vi "LineAlignment.vi"() -> ()   [LabVIEW 2018]
uses:
  <vilib>/Platform/TimedLoop/XDataNode/timing_clust.ctl
  <vilib>/Platform/TimedLoop/XDataNode/nitl_modes.ctl
  <vilib>/Platform/TimedLoop/XDataNode/wakeup.ctl
  LineAlignNotifier.ctl
  Drive/driveShifterEnum.ctl
  <userlib>/836-Library/System/TDMS_V2/Support/TDMS_DevRef.ctl
  <userlib>/836-Library/System/TDMS_V2/Support/Logging_Settings.ctl
  <userlib>/836-Library/System/TDMS_V2/Support/Group_FIFO_Config.ctl
  <userlib>/836-Library/System/TDMS_V2/Support/Channel_FIFO_Config.ctl
  <vilib>/addons/control/pid/pid.llb/PID (DBL).vi
  <vilib>/platform/TimedLoop/XDataNode/XDataNode.xnode
  <vilib>/addons/control/pid/NI_PID_pid.lvlib
  <vilib>/Platform/TimedLoop/XDataNode/XDNodeRunTimeDep.lvlib
panel:
  in  "Tab Control":enum32{"Auto Tape Alignment", "Drive PID Tune"}(tab)
  out "Chart":cluster{i16, i16, i16, "count":i32, "f":i32}(graph)={0, 0, 0, "count"=0, "f"=4}
  out "Late?":bool
  out "Arrived":bool=TRUE
  in  "Tol (in)":dbl=1.0
  in  "Tol (sec)":dbl=0.35 format="%#_13g"
  out "Right Front":bool
  out "Left Front":bool
  out "Right Rear":bool
  in  "PID gains":T1={"proportional gain (Kc)"=0.014, "integral time (Ti, min)"=0.02, "derivative time (Td, min)"=0.0001} {"derivative time (Td, min)" format="%.8f"; "integral time (Ti, min)" format="%.4f"; "proportional gain (Kc)" format="%.4f"}
  in  "clamp":cluster{"output high":dbl, "output low":dbl}={"output high"=1.0, "output low"=-1.0} {"output low" format="%.2f"; "output high" format="%.2f"}
  in  "Fwd offset Low":dbl=12.0
  in  "Rvs offset Low":dbl=12.0
  out "Goal":dbl=227.0788079155816
  out "Distance":dbl=227.1760531955295
  out "Tape Width":dbl=-5.971765136718773
  out "State":i32=4
  out "Error":dbl=-0.09724527994791288
  out "Count":i32
  out "Period":i64=10
  out "Left Rear":bool
  out "Fire Left":bool=TRUE
  out "Fire Right":bool
  in  "Push Drive":bool
  in  "Tune PID":bool
  in  "lo speed":dbl=0.4 format="%#_13g"
  in  "hi speed":dbl=0.75 format="%#_13g"
  in  "Avg Enc?":bool=TRUE
  in  "dead":dbl=0.05
  in  "Rvs offset High":dbl=12.0
  in  "Fwd offset High":dbl=12.0
  in  "Reset":bool
  in  "Rev":bool
  out "Align Assist":bool
  in  "Set":dbl(slide)=-0.07974481658691701 scale=-50.0..50.0
  in  "output range":cluster{"output high":dbl, "output low":dbl}={"output high"=0.65, "output low"=-0.65} {"output low" format="%.2f"; "output high" format="%.2f"}
  in  "PID gains 2":T1={"proportional gain (Kc)"=0.01, "integral time (Ti, min)"=0.01, "derivative time (Td, min)"=0.0001} {"derivative time (Td, min)" format="%.8f"; "integral time (Ti, min)" format="%.4f"; "proportional gain (Kc)" format="%.4f"}
  out "PID":cluster{"Set":dbl, "Distance":dbl}(graph)={"Set"=95.92025518341308, "Distance"=89.06027364430147}
  out "Error 2":dbl=6.859981539111601
  out "Motor":dbl=0.7000000000000001 format="%.2f"
  in  "reinit?":bool
  in  "negate":bool
  out "Arrived 2":bool
  in  "Tol (in) 2":dbl=0.75
  in  "Tol (sec) 2":dbl=0.35 format="%#_13g"
  out "Enc (in)":dbl=89.06027364430147
  out "Tuning":bool
  in  "Fwd":bool=TRUE
  out "Add":i32=96
  in  "dead 2":dbl=0.05
  in  "Reset Enc":bool
  # "old values;"
  # "Offset for Hi Gear = 21\"\nOffset for Lo Gear = 37\""
  # "Larger values move goal\nfurther in direction of travel"
  # "Diagnostics Only"
  # "Offset for Hi Gear = 12\"\nOffset for Lo Gear = 12\""
  # "2019 P-Bot Hi Gear values:\nP=0.0140, I=0.020, D=0.008"
  # "2019 P-Bot Lo Gear values:\nP=0.0, I=0.0, D=0.0"
  # "Initial 2019 Gear Set"
  # "2019 P-Bot Hi Gear values:\nP=0.0850, I=0.0090, D=0.000,000,08"
  # "2016 C-Bot Bot values:\nP=0.080, I=0.008, D=0.002"
  # "2019 P-Bot Lo Gear values:\nP=0.0350, I=0.0220, D=0.000,400"
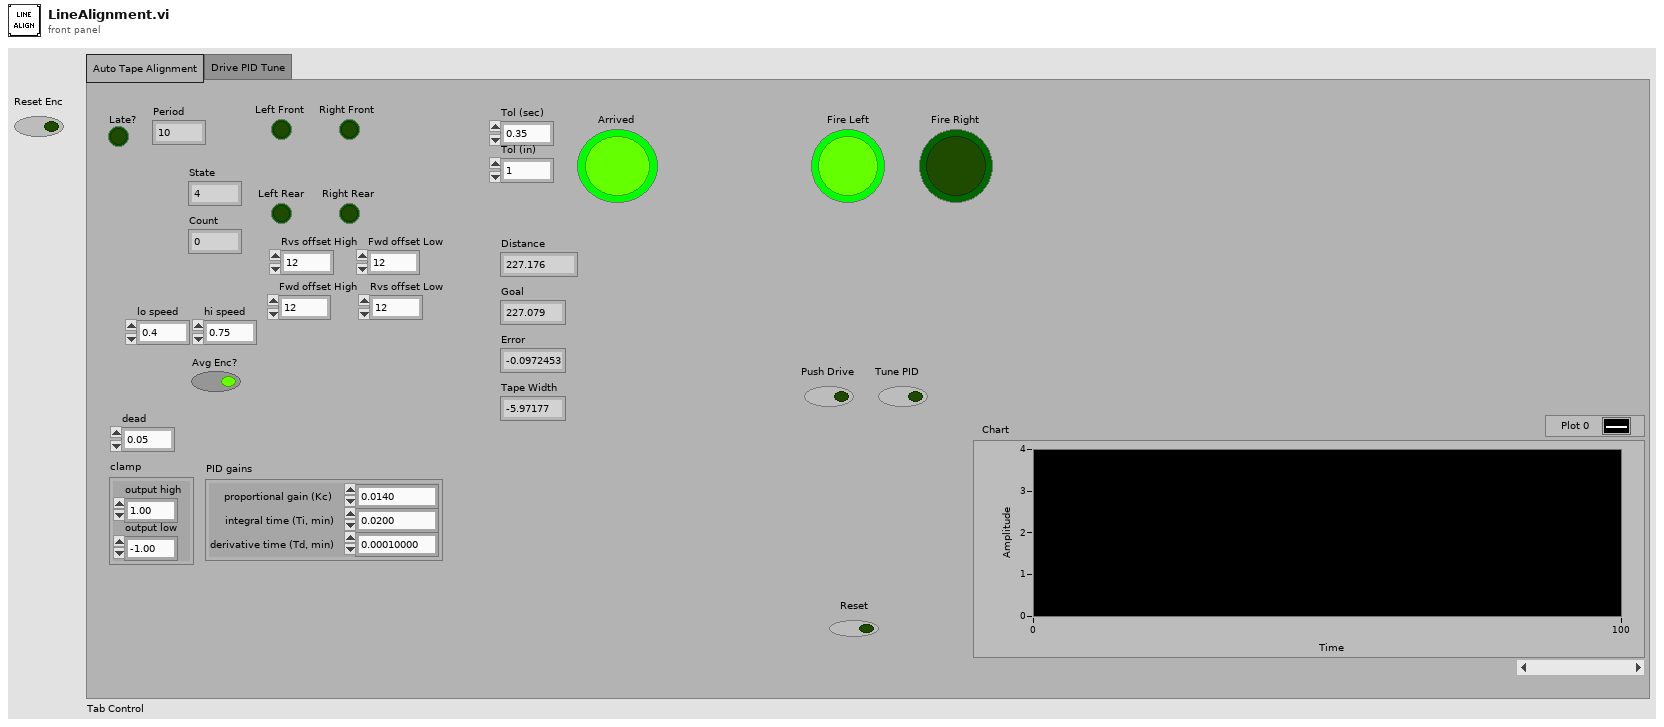
[diagram p1: front panel]
types:
  T1 = cluster{"proportional gain (Kc)":dbl, "integral time (Ti, min)":dbl, "derivative time (Td, min)":dbl}
  T2 = typedef "XDNodeRunTimeDep.lvlib/timing_clust.ctl" = cluster{"Expected End [f-1]":u64, "Actual End [f-1]":u64, "Finished Late? [f-1]":bool, "Expected End [i-1]":u64, "Actual End [i-1]":u64, "Finished Late? [i-1]":bool, "Expected Start [i]":u64, "Actual Start [i]":u64, "Expected Start [f]":u64, "Actual Start [f]":u64, "Source Name":string, "Structure Name":string, "Period":i64, "Deadline":i64, "Offset":i64, "Start":i64, "Priority":i32, "Timeout":i32, "Mode":T3, "Wakeup Reason":T4, "Error":errorcluster, "Source Type":string, "Secondary Source Type":string, "Global End Time":u64, "Global Start Time":u64, "Frame Duration":u64, "Iteration Duration":u64, "Assigned CPU":i32, "I/O Scan Engine Mode":u32}
  T3 = typedef "XDNodeRunTimeDep.lvlib/nitl_modes.ctl" = enum32{"No Change", "Process missed periods, maintain original phase", "Discard missed periods, maintain original phase", "Process missed periods, ignore original phase", "Discard missed periods, ignore original phase"}
  T4 = typedef "XDNodeRunTimeDep.lvlib/wakeup.ctl" = enum32{"Normal", "Aborted", "Asynchronous wakeup", "Timing source error", "Timed loop error", "Timeout"}
  T5 = typedef "driveShifterEnum.ctl" = enum16{"Low", "High"}
  T6 = typedef "LineAlignNotifier.ctl" = cluster{"skip 1":bool, "skip 2":bool, "LineAlign?":bool}
  T7 = typedef "TDMS_DevRef.ctl" = cluster{"Name":string, "File Ref":refnum<k34>, "Start Time":timestamp, "Logging Settings":T8, "Group FIFO Config":T9[], "Data To Write":refnum<data-value>, "semaphore":T11, "Ref Time Reset":refnum<k4>}
  T8 = typedef "Logging_Settings.ctl" = cluster{"Data Grab Period":dbl, "File Write Period":dbl, "Max Stored Size":dbl, "Burst Size":dbl}
  T9 = typedef "Group_FIFO_Config.ctl" = cluster{"Group":string, "Channels":T10[], "Channel Names":string[]}
  T10 = typedef "Channel_FIFO_Config.ctl" = cluster{"Channel":string, "FIFO":refnum<k33>}
  T11 = typedef "Semaphore RefNum" = refnum<k1>
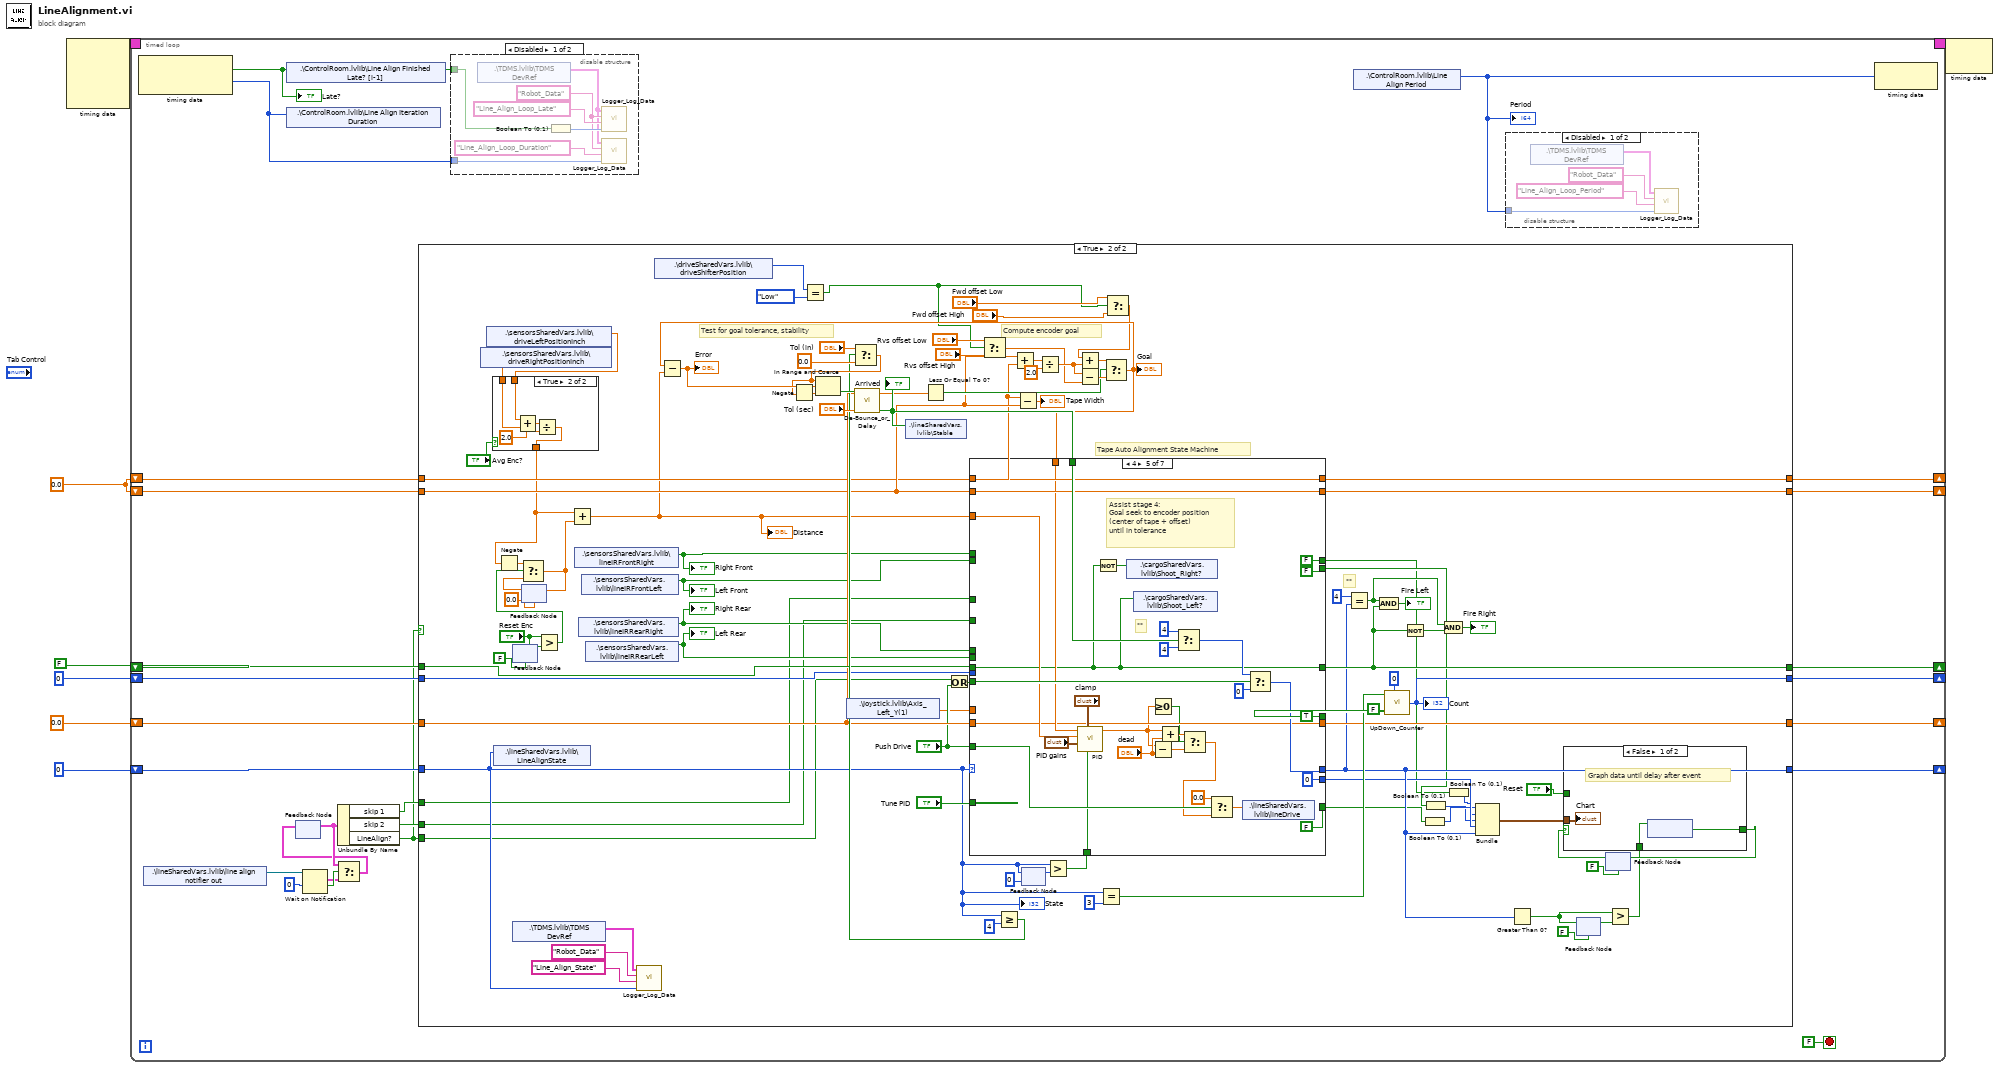
[diagram p0: block diagram]
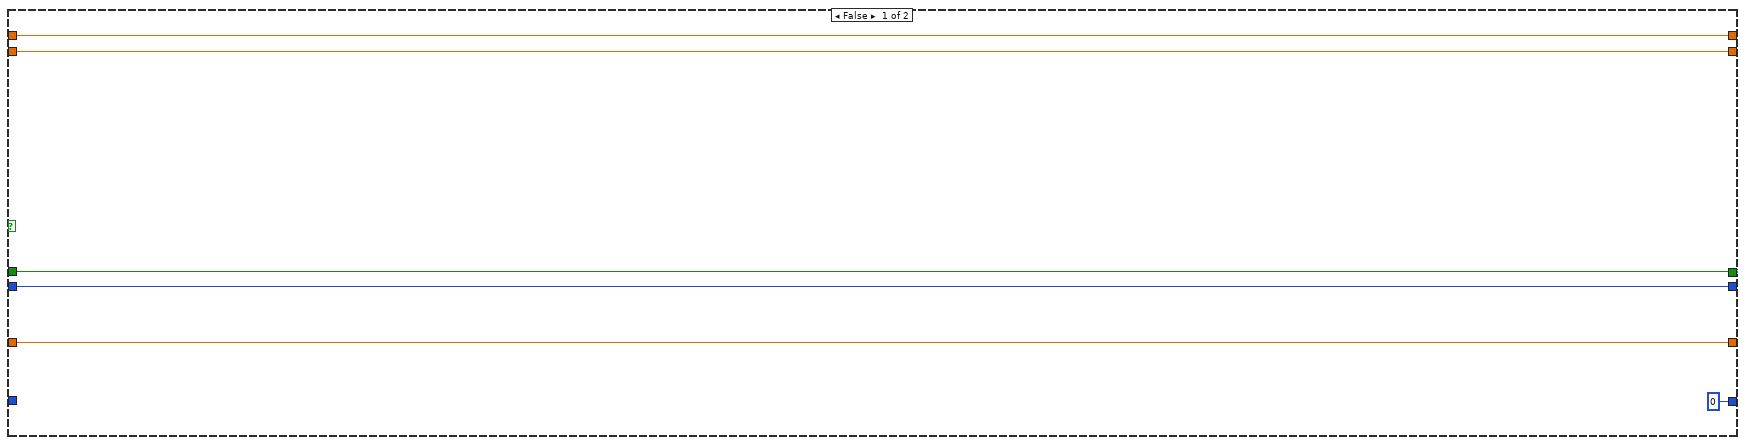
[diagram p2: hidden frame]
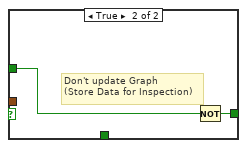
[diagram p3: hidden frame]
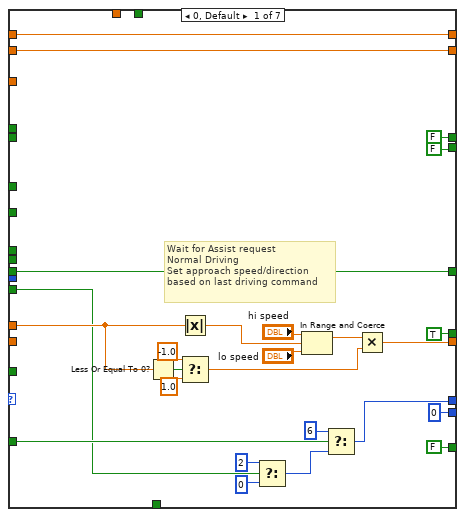
[diagram p5: hidden frame]
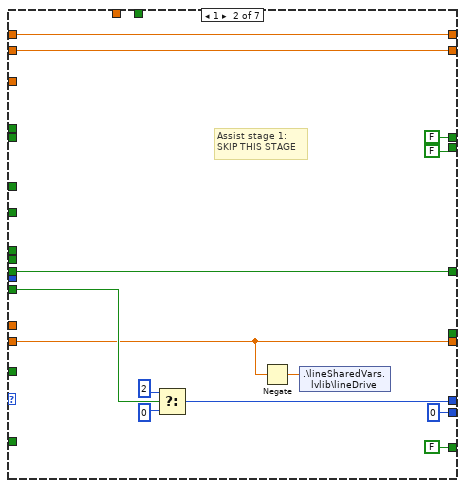
[diagram p6: hidden frame]
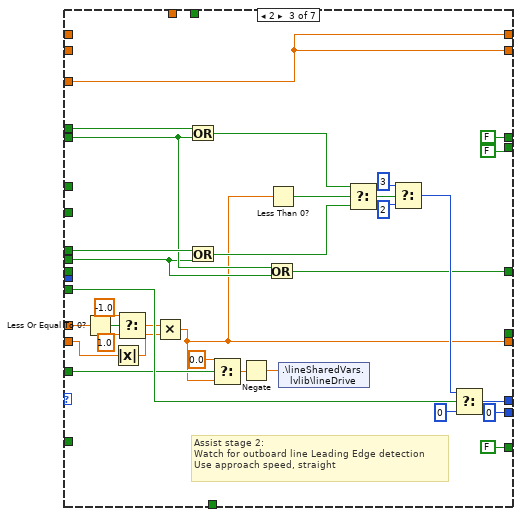
[diagram p7: hidden frame]
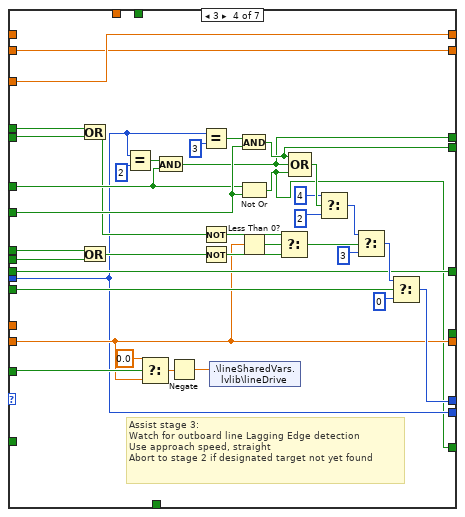
[diagram p8: hidden frame]
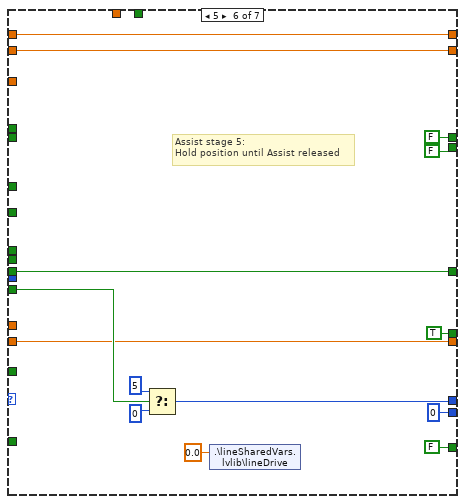
[diagram p9: hidden frame]
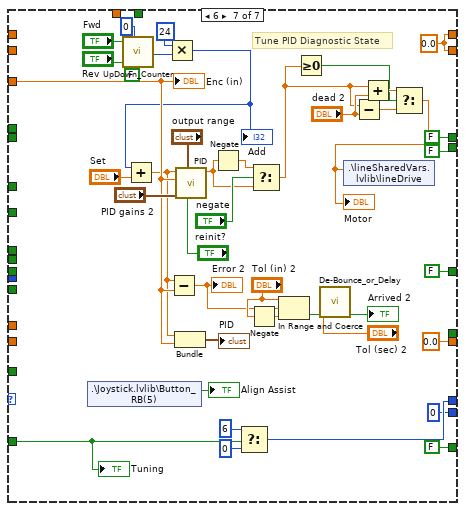
[diagram p10: hidden frame]
diagram:
  w1 = 0.0 ("Distance")
  n1 = node-c288() -> (w7:T2)  [unwired: 4 in]
  n2 = timed-loop {
    timing: w7 -> [_]
    timing-out: [_] -> w6
    shift-right: [w22] -> _
    shift-left: FALSE -> [w31]
    shift-right: [w30] -> _
    shift-left: 0.0 -> [w29]
    shift-right: [w21] -> _
    shift-left: 0 ("f") -> [w17]
    shift-right: [w28] -> _
    shift-left: 0 ("count") -> [w27]
    shift-right: [w26] -> _
    shift-left: w1 -> [w25]
    shift-right: [w24] -> _
    shift-left: w1 -> [w23]
    stop <- FALSE stop-if-true
    n3 = node-c288() -> (w20:bool, w19:i64)  [unwired: 1 in]
    "Late?" <- w20
    n4 = shared-variable ".\\lineSharedVars.lvlib\\line align notifier out"() -> (w12:refnum<notifier>)  [unwired: 1 in, 1 out]
    n5 = shared-variable ".\\ControlRoom.lvlib\\Line Align Finished Late? [i-1]"(w20) -> ()  [unwired: 1 in, 1 out]
    n6 = shared-variable ".\\ControlRoom.lvlib\\Line Align Iteration Duration"(w19) -> ()  [unwired: 1 in, 1 out]
    n7 = feedback #1() -> (w16:T6)  [unwired: 1 in]
    n8 = Wait on Notification(notifier=w12, timeout in ms (-1)=0) -> (notification=w14:T6, timed out?=w15:bool)  [unwired: 2 in, 2 out]
    n9 = Select(t=w16, s=w15, f=w14) -> (s? t:f=w9:T6)
    n10 = feedback-in #1(w9) -> ()
    n11 = Unbundle By Name(w16) -> ("skip 1"=w11:bool, "skip 2"=w10:bool, "LineAlign?"=w8:bool)
    n12 = case shown="True" w8 {
      tunnel: w31 -> [w36 w107]
      tunnel: [w38 w106] -> w30
      tunnel: w29 -> [w38 w105]
      tunnel: [w37 w104] -> w28
      tunnel: w27 -> [w37 w103]
      tunnel: [w35 w102] -> w26
      tunnel: w25 -> [w35 w101]
      tunnel: [w34 w100] -> w24
      tunnel: w23 -> [w34 w99]
      tunnel: [w36 w97] -> w22
      tunnel: [0 ("f") w56] -> w21
      tunnel: w17 -> [_ w48]
      tunnel: w11 -> [_ w47]
      tunnel: w10 -> [_ w46]
      tunnel: w8 -> [_ w45]
      frame False {
      }
      frame True {
        # "**"
        # "Tape Auto Alignment State Machine"
        # "Compute encoder goal"
        # "Test for goal tolerance, stability"
        n13 = shared-variable ".\\sensorsSharedVars.lvlib\\driveRightPositionInch"() -> (w72:dbl)  [unwired: 1 in, 1 out]
        n14 = shared-variable ".\\sensorsSharedVars.lvlib\\driveLeftPositionInch"() -> (w85:dbl)  [unwired: 1 in, 1 out]
        n15 = case shown="True" "Avg Enc?" {
          tunnel: w85 -> [w139 w144]
          tunnel: [w139 w141] -> w74
          tunnel: w72 -> [_ w140]
          frame False {
          }
          frame True {
            n16 = Add(x=w144, y=w140) -> (x+y=w143:dbl)
            n17 = Divide(x=w143, y=2.0) -> (x/y=w141:dbl)
          }
        }
        n18 = shared-variable ".\\lineSharedVars.lvlib\\LineAlignState"(w48) -> ()  [unwired: 1 in, 1 out]
        n19 = Negate(x=w74) -> (-x=w76:dbl)
        n20 = feedback #2(FALSE ("Reset Enc")) -> (w79:bool)
        n21 = feedback-in #2("Reset Enc") -> ()
        n22 = shared-variable ".\\TDMS.lvlib\\TDMS DevRef"() -> (w43:T7)  [unwired: 1 in, 1 out]
        n23 = feedback #3(0.0) -> (w84:dbl)
        n24 = Greater?(x="Reset Enc", y=w79) -> (0:w77:bool)
        n25 = Select(t=w76, s=w77, f=w84) -> (s? t:f=w82:dbl)
        n26 = feedback-in #3(w82) -> ()
        n27 = Add(x=w74, y=w82) -> (x+y=w81:dbl)
        "Distance" <- w81
        n28 = shared-variable ".\\sensorsSharedVars.lvlib\\lineIRFrontRight"() -> (w89:bool)  [unwired: 1 in, 1 out]
        "Right Front" <- w89
        n29 = shared-variable ".\\sensorsSharedVars.lvlib\\lineIRRearRight"() -> (w87:bool)  [unwired: 1 in, 1 out]
        "Right Rear" <- w87
        n30 = shared-variable ".\\sensorsSharedVars.lvlib\\lineIRFrontLeft"() -> (w88:bool)  [unwired: 1 in, 1 out]
        "Left Front" <- w88
        n31 = shared-variable ".\\sensorsSharedVars.lvlib\\lineIRRearLeft"() -> (w86:bool)  [unwired: 1 in, 1 out]
        "Left Rear" <- w86
        n32 = call <userlib>:"Logger_Log_Data.vi"("Data"=w48, "Channel"="Line_Align_State", "Group"="Robot_Data", "TDMS DevRef"=w43) -> ()  [unwired: 7 in, 1 out]
        n33 = shared-variable ".\\driveSharedVars.lvlib\\driveShifterPosition"() -> (w41:T5)  [unwired: 1 in, 1 out]
        n34 = Equal?(x=w41, y=driveShifterEnum."Low") -> (x = y?=w39:bool)
        n35 = shared-variable ".\\Joystick.lvlib\\Axis_Left_Y(1)"() -> (w75:dbl)  [unwired: 1 in, 1 out]
        n36 = Less Or Equal To 0?(x=w105) -> (x <= 0?=w114:bool)
        n37 = Or(x=w45, y="Push Drive") -> (x .or. y?=w91:bool)
        n38 = Select(t="Rvs offset Low", s=w39, f="Rvs offset High") -> (s? t:f=w68:dbl)
        n39 = Greater Or Equal?(x=w48, y=4) -> (x >= y?=w121:bool)
        n40 = Select(t="Tol (in)", s=w121, f=0.0 ("t")) -> (s? t:f=w125:dbl)
        n41 = Negate(x=w125) -> (-x=w132:dbl)
        n42 = Add(x=w101, y=w99) -> (x+y=w115:dbl)
        n43 = Subtract(x=w99, y=w101) -> (x-y=→"Tape Width":dbl)
        n44 = feedback #4(0) -> (w130:i32)
        n45 = feedback-in #4(w48) -> ()
        n46 = Divide(x=w115, y=2.0) -> (x/y=w117:dbl)
        n47 = Greater?(x=w48, y=w130) -> (0:w128:bool)
        n48 = Subtract(x=w117, y=w68) -> (x-y=w119:dbl)
        n49 = Equal?(x=w48, y=3) -> (x = y?=w109:bool)
        n50 = Select(t="Fwd offset Low", s=w39, f="Fwd offset High") -> (s? t:f=w70:dbl)
        n51 = Add(x=w70, y=w117) -> (x+y=w118:dbl)
        n52 = Select(t=w118, s=w114, f=w119) -> (s? t:f=w116:dbl)
        "Goal" <- w116
        n53 = Subtract(x=w116, y=w81) -> (x-y=w133:dbl)
        "Error" <- w133
        n54 = In Range and Coerce(upper limit=w125, x=w133, lower limit=w132) -> (In Range?=w127:bool)  [unwired: 1 out]
        n55 = call <userlib>:"De-Bounce_or_Delay.vi"("Eval Period (sec)"="Tol (sec)", "Signal Input"=w127) -> ("Stable"=w126:bool)  [unwired: 9 in]
        "Arrived" <- w126
        n56 = shared-variable ".\\lineSharedVars.lvlib\\Stable"(w126) -> ()  [unwired: 1 in, 1 out]
        n57 = case shown="4" w48 {
          tunnel: [w151 w182 w212 w249 w278 w293 w335] -> w56
          tunnel: w91 -> [w149 w181 w211 w251 w277 w296 _]
          tunnel: w75 -> [w157 _ w185 _ _ _ _]
          tunnel: [w162 w175 w186 w221 w261 w292 0.0] -> w106
          tunnel: w105 -> [_ w175 w183 w221 w261 w292 _]
          tunnel: w87 -> [_ _ w203 w230 _ _ _]
          tunnel: w89 -> [_ _ w205 w227 _ _ _]
          tunnel: w88 -> [_ _ w200 w226 _ _ _]
          tunnel: w81 -> [_ _ w208 w247 w275 _ w317]
          tunnel: [w167 w179 w208 w228 w273 w291 w318] -> w102
          tunnel: w101 -> [w167 w179 _ w228 w273 w291 _]
          tunnel: w126 -> [_ _ _ _ w274 _ _]
          tunnel: w128 -> [_ _ _ _ w267 _ _]
          tunnel: [w166 w178 w208 w247 w272 w290 w318] -> w100
          tunnel: w99 -> [w166 w178 _ _ w272 w290 _]
          tunnel: w116 -> [_ _ _ _ w271 _ _]
          tunnel: w47 -> [_ _ _ w240 _ _ _]
          tunnel: w46 -> [_ _ _ w241 _ _ _]
          tunnel: w103 -> [_ _ _ w218 _ _ _]
          tunnel: [TRUE _ _ _ TRUE TRUE _] -> w110
          tunnel: w86 -> [_ _ w199 w231 _ _ _]
          tunnel: [w154 w176 w201 w224 w257 w287 FALSE] -> w97
          tunnel: w107 -> [w154 w176 _ w224 w257 w287 _]
          tunnel: "Push Drive" -> [_ _ w197 w222 w268 _ _]
          tunnel: "Tune PID" -> [w150 _ _ _ _ _ w315]
          tunnel: [0 ("count") 0 ("count") 0 ("count") w218 0 ("count") 0 ("count") 0 ("count")] -> w55
          tunnel: [FALSE FALSE FALSE w217 FALSE FALSE FALSE] -> w51
          tunnel: [FALSE FALSE FALSE w216 FALSE FALSE FALSE] -> w49
          tunnel: [FALSE FALSE FALSE w215 FALSE FALSE FALSE] -> w54
          frame 0, Default {
            # "Wait for Assist request\nNormal Driving\nSet approach speed/direction\nbased on last driving command"
            n58 = Less Or Equal To 0?(x=w157) -> (x <= 0?=w161:bool)
            n59 = Absolute Value(x=w157) -> (abs(x)=w156:dbl)
            n60 = Select(t=-1.0, s=w161, f=1.0) -> (s? t:f=w158:dbl)
            n61 = Select(t=2, s=w149, f=0) -> (s? t:f=w153:i32)
            n62 = In Range and Coerce(upper limit="hi speed", x=w156, lower limit="lo speed") -> (coerced(x)=w163:dbl)  [unwired: 1 out]
            n63 = Select(t=6, s=w150, f=w153) -> (s? t:f=w151:i32)
            n64 = Multiply(x=w163, y=w158) -> (x*y=w162:dbl)
          }
          frame 1 {
            # "Assist stage 1:\nSKIP THIS STAGE"
            n65 = Select(t=2, s=w181, f=0) -> (s? t:f=w182:i32)
            n66 = Negate(x=w175) -> (-x=w174:dbl)
            n67 = shared-variable ".\\lineSharedVars.lvlib\\lineDrive"(w174) -> ()  [unwired: 1 in, 1 out]
          }
          frame 2 {
            # "Assist stage 2:\nWatch for outboard line Leading Edge detection\nUse approach speed, straight"
            n68 = Less Or Equal To 0?(x=w185) -> (x <= 0?=w190:bool)
            n69 = Absolute Value(x=w183) -> (abs(x)=w184:dbl)
            n70 = Select(t=-1.0, s=w190, f=1.0) -> (s? t:f=w187:dbl)
            n71 = Multiply(x=w187, y=w184) -> (x*y=w186:dbl)
            n72 = Or(x=w205, y=w200) -> (x .or. y?=w204:bool)
            n73 = Or(x=w203, y=w199) -> (x .or. y?=w202:bool)
            n74 = Select(t=0.0 ("Slow 2"), s=w197, f=w186) -> (s? t:f=w196:dbl)
            n75 = Negate(x=w196) -> (-x=w195:dbl)
            n76 = Or(x=w200, y=w199) -> (x .or. y?=w201:bool)
            n77 = Less Than 0?(x=w186) -> (x < 0?=w206:bool)
            n78 = shared-variable ".\\lineSharedVars.lvlib\\lineDrive"(w195) -> ()  [unwired: 1 in, 1 out]
            n79 = Select(t=w204, s=w206, f=w202) -> (s? t:f=w207:bool)
            n80 = Select(t=3 ("Jump"), s=w207, f=2) -> (s? t:f=w210:i32)
            n81 = Select(t=w210, s=w211, f=0) -> (s? t:f=w212:i32)
          }
          frame 3 {
            # "Assist stage 3:\nWatch for outboard line Lagging Edge detection\nUse approach speed, straight\nAbort to stage 2 if designated target not yet found"
            n82 = Or(x=w227, y=w226) -> (x .or. y?=w225:bool)
            n83 = Or(x=w230, y=w231) -> (x .or. y?=w229:bool)
            n84 = Equal?(x=w218, y=2) -> (x = y?=w246:bool)
            n85 = Select(t=0.0 ("Slow 2"), s=w222, f=w221) -> (s? t:f=w220:dbl)
            n86 = And(x=w246, y=w240) -> (x .and. y?=w216:bool)
            n87 = Negate(x=w220) -> (-x=w219:dbl)
            n88 = Equal?(x=w218, y=3) -> (x = y?=w243:bool)
            n89 = Not(x=w225) -> (.not. x?=w232:bool)
            n90 = Not(x=w229) -> (.not. x?=w233:bool)
            n91 = shared-variable ".\\lineSharedVars.lvlib\\lineDrive"(w219) -> ()  [unwired: 1 in, 1 out]
            n92 = And(x=w243, y=w241) -> (x .and. y?=w217:bool)
            n93 = Not Or(1:w241, 2:w240) -> (0:w215:bool)
            n94 = Less Than 0?(x=w221) -> (x < 0?=w235:bool)
            n95 = Select(t=w232, s=w235, f=w233) -> (s? t:f=w234:bool)
            n96 = Compound Arithmetic op=OR(w217, w216, w215) -> (w239:bool)
            n97 = Select(t=4, s=w239, f=2) -> (s? t:f=w238:i32)
            n98 = Select(t=w238, s=w234, f=3) -> (s? t:f=w237:i32)
            n99 = Select(t=w237, s=w251, f=0) -> (s? t:f=w249:i32)
          }
          frame 4 {
            # "**"
            # "Assist stage 4:\nGoal seek to encoder position\n(center of tape + offset)\nuntil in tolerance"
            n100 = call-poly <vilib>:"PID.vi"("reinitialize? (F)"=w267, "output range"="clamp", "PID gains"="PID gains", "process variable"=w275, "setpoint"=w271) -> ("output"=w259:dbl)  [unwired: 5 in, 1 out]
            n101 = Not(x=w257) -> (.not. x?=w258:bool)
            n102 = shared-variable ".\\cargoSharedVars.lvlib\\Shoot_Right?"(w258) -> ()  [unwired: 1 in, 1 out]
            n103 = shared-variable ".\\cargoSharedVars.lvlib\\Shoot_Left?"(w257) -> ()  [unwired: 1 in, 1 out]
            n104 = Greater Or Equal To 0?(x=w259) -> (x >= 0?=w260:bool)
            n105 = Subtract(x=w259, y="dead") -> (x-y=w264:dbl)
            n106 = Add(x=w259, y="dead") -> (x+y=w265:dbl)
            n107 = Select(t=4, s=w274, f=4) -> (s? t:f=w279:i32)
            n108 = Select(t=w265, s=w260, f=w264) -> (s? t:f=w263:dbl)
            n109 = Select(t=0.0 ("Slow 2"), s=w268, f=w263) -> (s? t:f=w266:dbl)
            n110 = shared-variable ".\\lineSharedVars.lvlib\\lineDrive"(w266) -> ()  [unwired: 1 in, 1 out]
            n111 = Select(t=w279, s=w277, f=0) -> (s? t:f=w278:i32)
          }
          frame 5 {
            # "Assist stage 5:\nHold position until Assist released"
            n112 = Select(t=5, s=w296, f=0) -> (s? t:f=w293:i32)
            n113 = shared-variable ".\\lineSharedVars.lvlib\\lineDrive"(0.0 ("Slow 2")) -> ()  [unwired: 1 in, 1 out]
          }
          frame 6 {
            w318 = 0.0 ("Distance")
            # "Tune PID Diagnostic State"
            n114 = shared-variable ".\\Joystick.lvlib\\Button_RB(5)"() -> (→"Align Assist":bool)  [unwired: 1 in, 1 out]
            n115 = call <userlib>:"UpDown_Counter.vi"("up"="Fwd", "initial"=0, "down"="Rev", "reset"=FALSE) -> ("count"=w312:i32)  [unwired: 1 in]
            n116 = Multiply(x=24, y=w312) -> (x*y=w309:i32)
            "Add" <- w309
            n117 = Add(x=w309, y="Set") -> (x+y=w310:dbl)
            n118 = Subtract(x=w310, y=w317) -> (x-y=w328:dbl)
            "Error 2" <- w328
            n119 = Bundle(w310, w317) -> (→"PID":cluster{dbl, dbl})  [unwired: 1 in]
            n120 = call-poly <vilib>:"PID.vi"("reinitialize? (F)"="reinit?", "output range"="output range", "PID gains"="PID gains 2", "process variable"=w317, "setpoint"=w310) -> ("output"=w323:dbl)  [unwired: 5 in, 1 out]
            n121 = Negate(x=w323) -> (-x=w324:dbl)
            n122 = Select(t=6, s=w315, f=0) -> (s? t:f=w335:i32)
            n123 = Negate(x="Tol (in) 2") -> (-x=w329:dbl)
            n124 = Select(t=w324, s="negate", f=w323) -> (s? t:f=w302:dbl)
            n125 = In Range and Coerce(upper limit="Tol (in) 2", x=w328, lower limit=w329) -> (In Range?=w331:bool)  [unwired: 1 out]
            n126 = Greater Or Equal To 0?(x=w302) -> (x >= 0?=w301:bool)
            n127 = call <userlib>:"De-Bounce_or_Delay.vi"("Eval Period (sec)"="Tol (sec) 2", "Signal Input"=w331) -> ("Stable"=→"Arrived 2":bool)  [unwired: 9 in]
            n128 = Subtract(x=w302, y="dead 2") -> (x-y=w305:dbl)
            n129 = Add(x=w302, y="dead 2") -> (x+y=w306:dbl)
            n130 = Select(t=w306, s=w301, f=w305) -> (s? t:f=w303:dbl)
            "Motor" <- w303
            n131 = shared-variable ".\\lineSharedVars.lvlib\\lineDrive"(w303) -> ()  [unwired: 1 in, 1 out]
            "Enc (in)" <- w317
            "Tuning" <- w315
          }
        }
        n132 = Equal?(x=4 ("y"), y=w56) -> (x = y?=w95:bool)
        n133 = And(x=w95, y=w97) -> (x .and. y?=→"Fire Left":bool)
        n134 = call <userlib>:"UpDown_Counter.vi"("up"=w109, "initial"=0, "down"=FALSE ("reset"), "reset"=w110) -> ("count"=w104:i32)  [unwired: 1 in]
        "Count" <- w104
        n135 = Not(x=w97) -> (.not. x?=w94:bool)
        n136 = Boolean To (0,1)(Boolean=w54) -> (0, 1=w53:i16)
        n137 = Boolean To (0,1)(Boolean=w51) -> (0, 1=w52:i16)
        n138 = And(x=w95, y=w94) -> (x .and. y?=→"Fire Right":bool)
        n139 = Boolean To (0,1)(Boolean=w49) -> (0, 1=w50:i16)
        n140 = Bundle(w53, w50, w52, "count"=w55, "f"=w56) -> (w57:cluster{i16, i16, i16, "count":i32, "f":i32})  [unwired: 1 in]
        n141 = Greater Than 0?(x=w56) -> (x > 0?=w58:bool)
        n142 = feedback #5(FALSE ("Shock")) -> (w62:bool)
        n143 = feedback-in #5(w58) -> ()
        n144 = feedback #6(FALSE) -> (w65:bool)
        n145 = Greater?(x=w58, y=w62) -> (0:w59:bool)
        n146 = case shown="False" w65 {
          tunnel: w59 -> [w136 _]
          tunnel: "Reset" -> [_ w137]
          tunnel: [w135 w138] -> w61
          tunnel: w57 -> [w134 _]
          frame False {
            # "Graph data until delay after event"
            n147 = feedback #7() -> (w135:bool)  [unwired: 1 in]
            n148 = feedback-in #7(w136) -> ()
            "Chart" <- w134
          }
          frame True {
            # "Don't update Graph\n(Store Data for Inspection)"
            n149 = Not(x=w137) -> (.not. x?=w138:bool)
          }
        }
        n150 = feedback-in #6(w61) -> ()
        "State" <- w48
      }
    }
    n151 = disable-structure shown="Disabled" {
      disable-tunnel: w20 -> [w339 _]
      disable-tunnel: w19 -> [w338 _]
      frame Disabled {
        w341 = "Robot_Data" ("Group")
        n152 = shared-variable ".\\TDMS.lvlib\\TDMS DevRef"() -> (w340:T7)  [unwired: 1 in, 1 out]
        n153 = Boolean To (0,1)(Boolean=w339) -> (0, 1=w343:i16)
        n154 = call <userlib>:"Logger_Log_Data.vi"("Data"=w343, "Channel"="Line_Align_Loop_Late", "Group"=w341, "TDMS DevRef"=w340) -> ()  [unwired: 7 in, 1 out]
        n155 = call <userlib>:"Logger_Log_Data.vi"("Data"=w338, "Channel"="Line_Align_Loop_Duration", "Group"=w341, "TDMS DevRef"=w340) -> ()  [unwired: 7 in, 1 out]
      }
      frame Enabled {
      }
    }
    n156 = shared-variable ".\\ControlRoom.lvlib\\Line Align Period"() -> (w18:i64)  [unwired: 1 in, 1 out]
    "Period" <- w18
    n157 = disable-structure shown="Disabled" {
      disable-tunnel: w18 -> [w345 _]
      frame Disabled {
        n158 = shared-variable ".\\TDMS.lvlib\\TDMS DevRef"() -> (w347:T7)  [unwired: 1 in, 1 out]
        n159 = call <userlib>:"Logger_Log_Data.vi"("Data"=w345, "Channel"="Line_Align_Loop_Period", "Group"="Robot_Data", "TDMS DevRef"=w347) -> ()  [unwired: 7 in, 1 out]
      }
      frame Enabled {
      }
    }
    n160 = node-c288(w18) -> ()  [unwired: 1 out]
  }
  n161 = node-c288(w6) -> ()  [unwired: 1 out]
